vi "GET_Statistics_(online).vi"(0 "Animal coordinates in":T6 {"Measurements and statistics"."Running, perc. of time" format="%05.2f"}, 2 "Stats parameters (online)":T2={"Mouse drawing parameters"={"Trace length, samples"=0, "Rainbow track"=FALSE, "Rainbow track is speed"=FALSE, "Bright mouse lineout"=FALSE, "Colors array"=[], "Pixels per mm"=0.0}, "Size of the image (480x480)"={"Numeric Control"=480.0, "Numeric Control"=480.0}, "Array of the pixel to zone correspondences"=[], "Hist. bins array"=[], "Histogram parameters"={"max"=300.0, "min"=0.0, "# bins"=10, "threshold"=8.0, "thr. type"=enum."higher accepted"}}, 3 "Reset? (F)":bool, 5 "error in (no error)":T1) -> (6 "Animal coordinates out":T6 {"Measurements and statistics"."Running, perc. of time" format="%05.2f"}, 8 "error out":T1)   [LabVIEW 2018, in "Tracker.lvlib"]
uses:
  Tracker.lvlib
  Controls/CTL_Full_data_frame.ctl
  Controls/CTL_Animal_Coordinates_and_Speed.ctl
  Controls/CTL_Measurements_and_Statistics.ctl
  Controls/CTL_Stats_parameters_(online).ctl
  Controls/CTL_Mouse_Draw_Params.ctl
  Controls/CTL_Pixel_to_Zone_array.ctl
  Controls/CTL_Histogram_parameters.ctl
  Common_Resources.lvlib
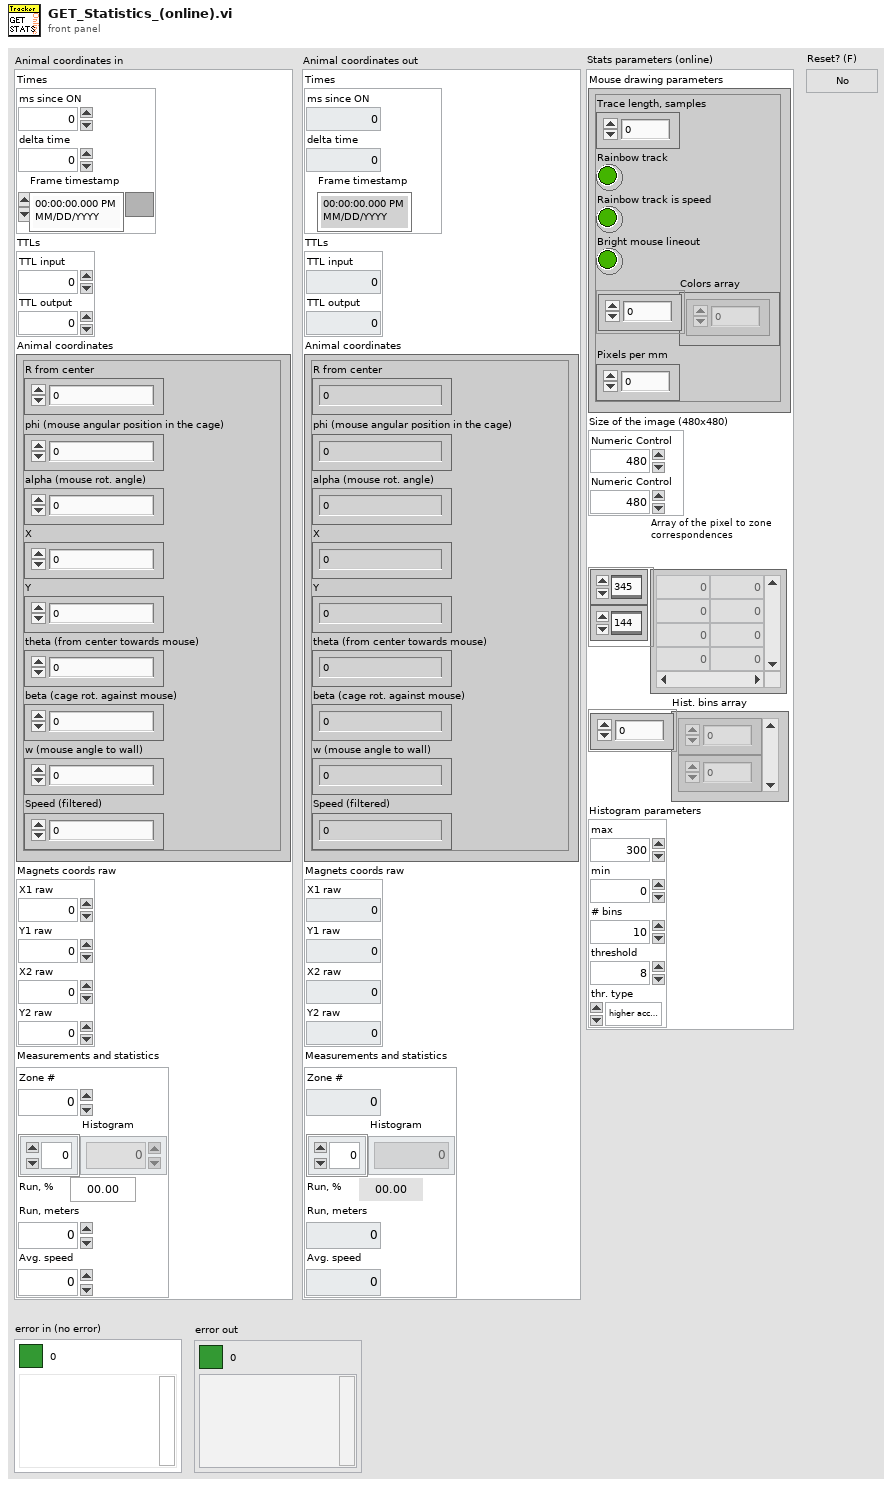
[diagram p1: front panel]
types:
  T1 = cluster{"Boolean Round":bool, "code":i32, "source":string}
  T2 = typedef "Common_Resources.lvlib/CTL_Stats_parameters_(online).ctl" = cluster{"Mouse drawing parameters":T3, "Size of the image (480x480)":cluster{"Numeric Control":dbl, "Numeric Control":dbl}, "Array of the pixel to zone correspondences":T4, "Hist. bins array":dbl[], "Histogram parameters":T5}
  T3 = typedef "Common_Resources.lvlib/CTL_Mouse_Draw_Params.ctl" = cluster{"Trace length, samples":u16, "Rainbow track":bool, "Rainbow track is speed":bool, "Bright mouse lineout":bool, "Colors array":u32[], "Pixels per mm":dbl}
  T4 = typedef "Common_Resources.lvlib/CTL_Pixel_to_Zone_array.ctl" = i8[][]
  T5 = typedef "Common_Resources.lvlib/CTL_Histogram_parameters.ctl" = cluster{"max":dbl, "min":dbl, "# bins":i32, "threshold":dbl, "thr. type":enum16{"higher accepted", "lower accepted"}}
  T6 = typedef "Common_Resources.lvlib/CTL_Full_data_frame.ctl" = cluster{"Times":cluster{"ms since ON":u32, "delta time":u32, "Frame timestamp":timestamp}, "TTLs":cluster{"TTL input":i16, "TTL output":i16}, "Animal coordinates":T7, "Magnets coords raw":cluster{"X1 raw":dbl, "Y1 raw":dbl, "X2 raw":dbl, "Y2 raw":dbl}, "Measurements and statistics":T8}
  T7 = typedef "Common_Resources.lvlib/CTL_Animal_Coordinates_and_Speed.ctl" = cluster{"R from center":dbl, "phi (mouse angular position in the cage)":dbl, "alpha (mouse rot. angle)":dbl, "X":dbl, "Y":dbl, "theta (from center towards mouse)":dbl, "beta (cage rot. against mouse)":dbl, "w (mouse angle to wall)":dbl, "Speed (filtered)":dbl}
  T8 = typedef "Common_Resources.lvlib/CTL_Measurements_and_Statistics.ctl" = cluster{"Zone #":i8, "Histogram":dbl[], "Running, perc. of time":dbl, "Run, meters":dbl, "Avg. speed":dbl}
  T9 = cluster{"Numeric Control":dbl, "Numeric Control":dbl}
  T10 = typedef "Common_Resources.lvlib/CTL_Running_statistics_results.ctl" = cluster{"Thresholded":u32, "Total":u32, "Percentage":dbl, "Run, meters":dbl, "Avg. speed":dbl}
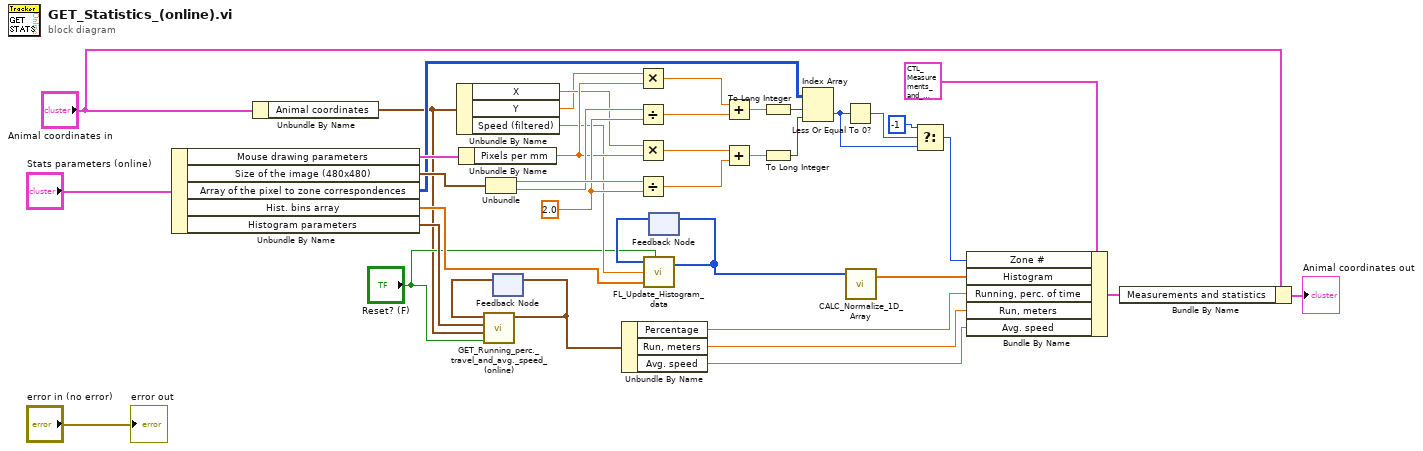
[diagram p0: block diagram]
diagram:
  w38 = 2.0
  n1 = Unbundle By Name("Stats parameters (online)") -> ("Mouse drawing parameters"=w19:T3, "Size of the image (480x480)"=w18:T9, "Array of the pixel to zone correspondences"=w17:T4, "Hist. bins array"=w16:dbl[], "Histogram parameters"=w15:T5)
  n2 = Unbundle By Name("Animal coordinates in") -> ("Animal coordinates"=w5:T7)
  n3 = Unbundle By Name(w5) -> ("X"=w9:dbl, "Y"=w8:dbl, "Speed (filtered)"=w14:dbl)
  n4 = Unbundle By Name(w19) -> ("Pixels per mm"=w35:dbl)
  n5 = Unbundle(w18) -> ("Numeric Control"=w40:dbl, "Numeric Control"=w39:dbl)
  n6 = feedback #1() -> (w12:T10)  [unwired: 1 in]
  n7 = call "GET_Running_perc._travel_and_avg._speed_(online).vi"("Reset? (F)"="Reset? (F)", "Animal coordinates in"=w5, "Histogram parameters"=w15, "Running stats results in"=w12) -> ("Running stats results out"=w11:T10)  [unwired: 7 in]
  n8 = feedback-in #1(w11) -> ()
  n9 = Unbundle By Name(w11) -> ("Percentage"=w10:dbl, "Run, meters"=w7:dbl, "Avg. speed"=w1:dbl)
  n10 = Multiply(x=w8, y=w35) -> (x*y=w33:dbl)
  n11 = Divide(x=w39, y=w38) -> (x/y=w36:dbl)
  n12 = Multiply(x=w9, y=w35) -> (x*y=w34:dbl)
  n13 = Divide(x=w40, y=w38) -> (x/y=w37:dbl)
  n14 = feedback #2() -> (w24:u32[])  [unwired: 1 in]
  n15 = call "FL_Update_Histogram_data.vi"("Histogram count in"=w24, "Reset? (F)"="Reset? (F)", "Current value"=w14, "Bins array"=w16) -> ("Histogram count out"=w25:u32[])  [unwired: 2 in]
  n16 = feedback-in #2(w25) -> ()
  n17 = Add(x=w33, y=w36) -> (x+y=w31:dbl)
  n18 = Add(x=w34, y=w37) -> (x+y=w32:dbl)
  n19 = To Long Integer(number=w31) -> (32bit integer=w29:i32)
  n20 = To Long Integer(number=w32) -> (32bit integer=w30:i32)
  n21 = Index Array(array=w17, index (row)=w29, index (col)=w30) -> (element=w26:i8)
  n22 = Less Or Equal To 0?(x=w26) -> (x <= 0?=w28:bool)
  n23 = call "CALC_Normalize_1D_Array.vi"("1D array"=w25) -> ("Normalized 1D array"=w22:dbl[])  [unwired: 2 in, 1 out]
  n24 = Select(t=i8 -1, s=w28, f=w26) -> (s? t:f=w23:i8)
  n25 = Bundle By Name(cluster=T8 {"Zone #"=0, "Histogram"=[], "Running, perc. of time"=0.28949046360238656, "Run, meters"=0.0, "Avg. speed"=0.0} ("Measurements and statistics"), "Zone #"=w23, "Histogram"=w22, "Running, perc. of time"=w10, "Run, meters"=w7, "Avg. speed"=w1) -> (w3:T8)
  n26 = Bundle By Name(cluster="Animal coordinates in", "Measurements and statistics"=w3) -> (→"Animal coordinates out":T6)
  "error out" <- "error in (no error)"
